vi "Delay.vi"(7 "대기시간 (초)":dbl, 8 "error in":errorcluster caption="에러 입력(에러 없음)", 9 "정지?":bool) -> (0 "error out":errorcluster caption="에러 출력", 3 "Elapsed Time (s)":dbl caption="경과 시간(초)")   [LabVIEW 2020]
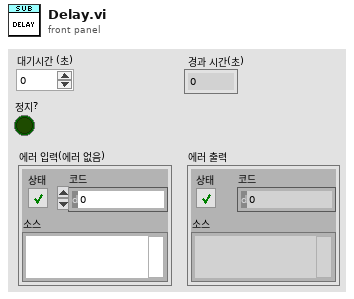
[diagram p1: front panel]
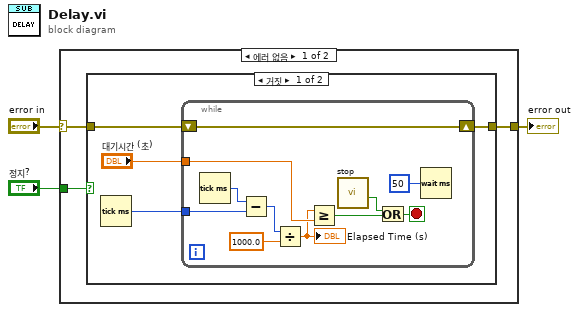
[diagram p0: block diagram]
diagram:
  n1 = case shown="에러 없음" "error in" {
    selector: "error in" -> [w5 w23]
    tunnel: [w4 w23] -> w1
    tunnel: "정지?" -> [w6 _]
    frame No Error {
      n2 = case shown="거짓" w6 {
        tunnel: w5 -> [w9 w22]
        tunnel: [w8 w22] -> w4
        frame False {
          n3 = Tick Count (ms)() -> (millisecond timer value=w7:u32)
          n4 = while {
            tunnel: "대기시간 (초)" -> [w17]
            shift-right: [w18] -> w8
            shift-left: w9 -> [w18]
            tunnel: w7 -> [w14]
            stop <- w20 stop-if-true
            n5 = Tick Count (ms)() -> (millisecond timer value=w15:u32)
            n6 = Subtract(x=w15, y=w14) -> (x-y=w13:u32)
            n7 = Divide(x=w13, y=1000.0) -> (x/y=w11:dbl)
            "Elapsed Time (s)" <- w11
            n8 = Greater Or Equal?(x=w11, y=w17) -> (x >= y?=w16:bool)
            n9 = call "stop.vi"() -> ("stop?"=w19:bool)  [unwired: 10 in, 1 out]
            n10 = Or(x=w19, y=w16) -> (x .or. y?=w20:bool)
            n11 = Wait (ms)(milliseconds to wait=u32 50 ("대기 시간(ms)")) -> ()  [unwired: 1 out]
          }
        }
        frame True {
        }
      }
    }
    frame Error {
    }
  }
  "error out" <- w1
